vi "Ex2_Serrure_Num.vi"() -> ()   [LabVIEW 2018]
panel:
  out "Boolean":bool
  in  "2":u8(knob) scale=0.0..9.0
  in  "1":u8(knob) scale=0.0..9.0
  in  "3":u8(knob) scale=0.0..9.0
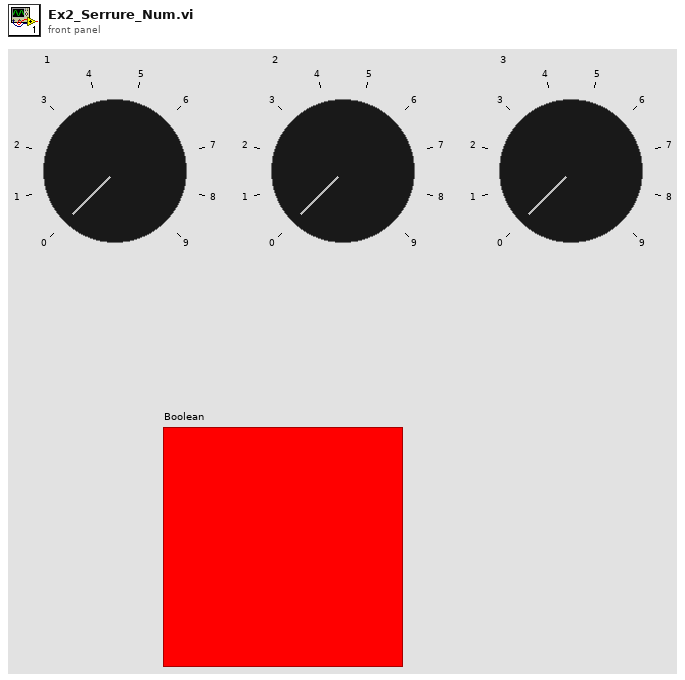
[diagram p1: front panel]
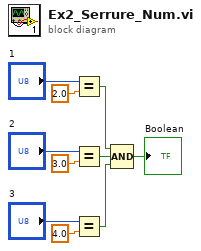
[diagram p0: block diagram]
diagram:
  n1 = Equal?(x="1", y=2.0 ("2")) -> (x = y?=w4:bool)
  n2 = Equal?(x="2", y=3.0 ("2")) -> (x = y?=w3:bool)
  n3 = Equal?(x="3", y=4.0 ("2")) -> (x = y?=w2:bool)
  n4 = Compound Arithmetic op=AND(w4, w3, w2) -> (→"Boolean":bool)
